vi "OCR Player2 DeleteMe.vi"(7 "error in":errorcluster) -> (27 "error out":errorcluster)   [LabVIEW 2015]
uses:
  <vilib>/vision/NI_Vision_Development_Module.lvlib
panel:
  out "Image Out":T1(plugin-control)
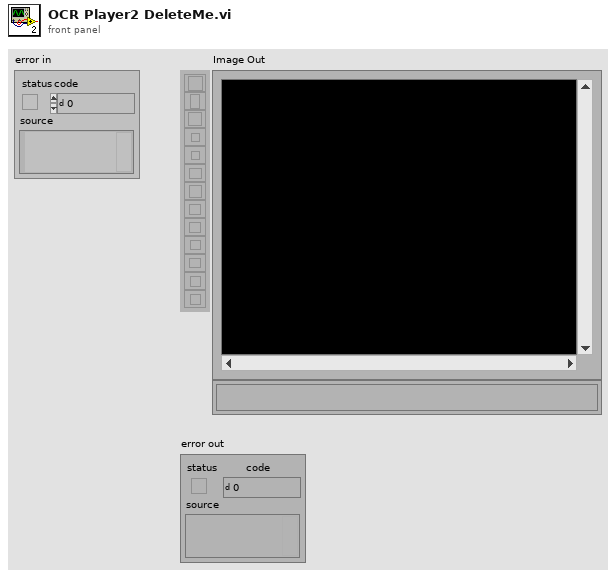
[diagram p1: front panel]
types:
  T1 = typedef "IMAQ Image.ctl" = refnum<image>
  T2 = cluster{"Threshold Data":cluster{"Method":enum16{"Fixed Range", "Uniform", "Linear", "Non Linear", "Local", "Color"}, "Looking for":u32, "Color Mode":u32, "Kernel Size":cluster{"Width":i32, "Height":i32}, "Ranges":cluster{"Min":i32, "Max":i32}[]}, "Reject Border":bool, "Number Of Erosions":i32, "Size & Spacing":cluster{"Segment Algorithm":u16, "Min Bounding Rect Width":i32, "Max Bounding Rect Width":i32, "Min Bounding Rect Height":i32, "Max Bounding Rect Height":i32, "Min Character Size":i32, "Max Character Size":i32, "Min Char Spacing":i32, "Max Horiz Element Spacing":i32, "Max Vert Element Spacing":i32, "Max Space Distance":i32}, "Read Options":cluster{"Read Strategy":i32, "Read Resolution":i32, "Scale Dependant":bool, "Aspect Ratio":i32, "Acceptance Level":i32, "Substitution Character":string, "MultiLine":bool}, "Valid Characters":cluster{"Pre-defined characters":i32, "User-defined characters":string}[], "Use Text Pattern":bool, "Orientation":u32, "# Lines Expected":u32, "Number of Blocks":i32}
  T3 = cluster{"Global Rectangle":i32[], "Contours":cluster{"ID":enum32{"External", "Internal"}, "Type":u32, "Coordinates":i32[]}[]}
  T4 = typedef "Image Type" = u32
  T5 = typedef "IMAQ OCR Session.ctl" = refnum<k1>
diagram:
  w1 = u32 0 items=["Grayscale", "Binary", "Gradient", "Rainbow", "Temperature", "User Defined", "Binary 16 Bit", "Gradient 16 Bit", "Rainbow 16 Bit", "Temperature 16 Bit", "User Defined 16 Bit"] ("Palette Type")
  w10 = T2 {"Threshold Data"={"Method"=enum."Uniform", "Looking for"=1, "Color Mode"=0, "Kernel Size"={"Width"=32, "Height"=32}, "Ranges"=[{"Min"=1, "Max"=255}]}, "Reject Border"=TRUE, "Number Of Erosions"=0, "Size & Spacing"={"Segment Algorithm"=0, "Min Bounding Rect Width"=2, "Max Bounding Rect Width"=8, "Min Bounding Rect Height"=2, "Max Bounding Rect Height"=65536, "Min Character Size"=4, "Max Character Size"=5555, "Min Char Spacing"=1, "Max Horiz Element Spacing"=1, "Max Vert Element Spacing"=0, "Max Space Distance"=65536}, "Read Options"={"Read Strategy"=1, "Read Resolution"=2, "Scale Dependant"=FALSE, "Aspect Ratio"=400, "Acceptance Level"=700, "Substitution Character"="?", "MultiLine"=FALSE}, "Valid Characters"=[], "Use Text Pattern"=FALSE, "Orientation"=0, "# Lines Expected"=0, "Number of Blocks"=4}  # Parameters
  w11 = T3 {"Global Rectangle"=[720, 494, 833, 510], "Contours"=[{"ID"=enum."External", "Type"=3, "Coordinates"=[720, 494, 833, 510]}]}  # ROI Descriptor
  w19 = T2 {"Threshold Data"={"Method"=enum."Uniform", "Looking for"=1, "Color Mode"=0, "Kernel Size"={"Width"=32, "Height"=32}, "Ranges"=[{"Min"=1, "Max"=255}]}, "Reject Border"=TRUE, "Number Of Erosions"=0, "Size & Spacing"={"Segment Algorithm"=0, "Min Bounding Rect Width"=2, "Max Bounding Rect Width"=8, "Min Bounding Rect Height"=2, "Max Bounding Rect Height"=65536, "Min Character Size"=4, "Max Character Size"=5555, "Min Char Spacing"=1, "Max Horiz Element Spacing"=1, "Max Vert Element Spacing"=0, "Max Space Distance"=65536}, "Read Options"={"Read Strategy"=1, "Read Resolution"=2, "Scale Dependant"=FALSE, "Aspect Ratio"=400, "Acceptance Level"=700, "Substitution Character"="?", "MultiLine"=FALSE}, "Valid Characters"=[], "Use Text Pattern"=FALSE, "Orientation"=0, "# Lines Expected"=0, "Number of Blocks"=4}  # Parameters
  w20 = T3 {"Global Rectangle"=[523, 533, 645, 550], "Contours"=[{"ID"=enum."External", "Type"=3, "Coordinates"=[523, 533, 645, 550]}]}  # ROI Descriptor
  w28 = T2 {"Threshold Data"={"Method"=enum."Uniform", "Looking for"=1, "Color Mode"=0, "Kernel Size"={"Width"=32, "Height"=32}, "Ranges"=[{"Min"=1, "Max"=255}]}, "Reject Border"=TRUE, "Number Of Erosions"=0, "Size & Spacing"={"Segment Algorithm"=0, "Min Bounding Rect Width"=2, "Max Bounding Rect Width"=8, "Min Bounding Rect Height"=2, "Max Bounding Rect Height"=65536, "Min Character Size"=4, "Max Character Size"=5555, "Min Char Spacing"=1, "Max Horiz Element Spacing"=1, "Max Vert Element Spacing"=0, "Max Space Distance"=65536}, "Read Options"={"Read Strategy"=1, "Read Resolution"=2, "Scale Dependant"=FALSE, "Aspect Ratio"=400, "Acceptance Level"=700, "Substitution Character"="?", "MultiLine"=FALSE}, "Valid Characters"=[], "Use Text Pattern"=FALSE, "Orientation"=0, "# Lines Expected"=0, "Number of Blocks"=4}  # Parameters
  w29 = T3 {"Global Rectangle"=[386, 689, 502, 706], "Contours"=[{"ID"=enum."External", "Type"=3, "Coordinates"=[386, 689, 502, 706]}]}  # ROI Descriptor
  w37 = T2 {"Threshold Data"={"Method"=enum."Uniform", "Looking for"=1, "Color Mode"=0, "Kernel Size"={"Width"=32, "Height"=32}, "Ranges"=[{"Min"=1, "Max"=255}]}, "Reject Border"=TRUE, "Number Of Erosions"=0, "Size & Spacing"={"Segment Algorithm"=0, "Min Bounding Rect Width"=2, "Max Bounding Rect Width"=8, "Min Bounding Rect Height"=2, "Max Bounding Rect Height"=65536, "Min Character Size"=4, "Max Character Size"=5555, "Min Char Spacing"=1, "Max Horiz Element Spacing"=1, "Max Vert Element Spacing"=0, "Max Space Distance"=65536}, "Read Options"={"Read Strategy"=1, "Read Resolution"=2, "Scale Dependant"=FALSE, "Aspect Ratio"=400, "Acceptance Level"=700, "Substitution Character"="?", "MultiLine"=FALSE}, "Valid Characters"=[], "Use Text Pattern"=FALSE, "Orientation"=0, "# Lines Expected"=0, "Number of Blocks"=4}  # Parameters
  w38 = T3 {"Global Rectangle"=[543, 836, 661, 852], "Contours"=[{"ID"=enum."External", "Type"=3, "Coordinates"=[543, 836, 661, 852]}]}  # ROI Descriptor
  w46 = T2 {"Threshold Data"={"Method"=enum."Uniform", "Looking for"=1, "Color Mode"=0, "Kernel Size"={"Width"=32, "Height"=32}, "Ranges"=[{"Min"=1, "Max"=255}]}, "Reject Border"=TRUE, "Number Of Erosions"=0, "Size & Spacing"={"Segment Algorithm"=0, "Min Bounding Rect Width"=2, "Max Bounding Rect Width"=8, "Min Bounding Rect Height"=2, "Max Bounding Rect Height"=65536, "Min Character Size"=4, "Max Character Size"=5555, "Min Char Spacing"=1, "Max Horiz Element Spacing"=1, "Max Vert Element Spacing"=0, "Max Space Distance"=65536}, "Read Options"={"Read Strategy"=1, "Read Resolution"=2, "Scale Dependant"=FALSE, "Aspect Ratio"=400, "Acceptance Level"=700, "Substitution Character"="?", "MultiLine"=FALSE}, "Valid Characters"=[], "Use Text Pattern"=FALSE, "Orientation"=0, "# Lines Expected"=0, "Number of Blocks"=4}  # Parameters
  w47 = T3 {"Global Rectangle"=[757, 870, 877, 885], "Contours"=[{"ID"=enum."External", "Type"=3, "Coordinates"=[757, 870, 877, 885]}]}  # ROI Descriptor
  w55 = T2 {"Threshold Data"={"Method"=enum."Uniform", "Looking for"=1, "Color Mode"=0, "Kernel Size"={"Width"=32, "Height"=32}, "Ranges"=[{"Min"=1, "Max"=255}]}, "Reject Border"=TRUE, "Number Of Erosions"=0, "Size & Spacing"={"Segment Algorithm"=0, "Min Bounding Rect Width"=2, "Max Bounding Rect Width"=8, "Min Bounding Rect Height"=2, "Max Bounding Rect Height"=65536, "Min Character Size"=4, "Max Character Size"=5555, "Min Char Spacing"=1, "Max Horiz Element Spacing"=1, "Max Vert Element Spacing"=0, "Max Space Distance"=65536}, "Read Options"={"Read Strategy"=1, "Read Resolution"=2, "Scale Dependant"=FALSE, "Aspect Ratio"=400, "Acceptance Level"=700, "Substitution Character"="?", "MultiLine"=FALSE}, "Valid Characters"=[], "Use Text Pattern"=FALSE, "Orientation"=0, "# Lines Expected"=0, "Number of Blocks"=4}  # Parameters
  w56 = T3 {"Global Rectangle"=[1029, 868, 1143, 884], "Contours"=[{"ID"=enum."External", "Type"=3, "Coordinates"=[1029, 868, 1143, 884]}]}  # ROI Descriptor
  w64 = T2 {"Threshold Data"={"Method"=enum."Uniform", "Looking for"=1, "Color Mode"=0, "Kernel Size"={"Width"=32, "Height"=32}, "Ranges"=[{"Min"=1, "Max"=255}]}, "Reject Border"=TRUE, "Number Of Erosions"=0, "Size & Spacing"={"Segment Algorithm"=0, "Min Bounding Rect Width"=2, "Max Bounding Rect Width"=8, "Min Bounding Rect Height"=2, "Max Bounding Rect Height"=65536, "Min Character Size"=4, "Max Character Size"=5555, "Min Char Spacing"=1, "Max Horiz Element Spacing"=1, "Max Vert Element Spacing"=0, "Max Space Distance"=65536}, "Read Options"={"Read Strategy"=1, "Read Resolution"=2, "Scale Dependant"=FALSE, "Aspect Ratio"=400, "Acceptance Level"=700, "Substitution Character"="?", "MultiLine"=FALSE}, "Valid Characters"=[], "Use Text Pattern"=FALSE, "Orientation"=0, "# Lines Expected"=0, "Number of Blocks"=4}  # Parameters
  w65 = T3 {"Global Rectangle"=[1264, 838, 1374, 853], "Contours"=[{"ID"=enum."External", "Type"=3, "Coordinates"=[1264, 838, 1374, 853]}]}  # ROI Descriptor
  w73 = T2 {"Threshold Data"={"Method"=enum."Uniform", "Looking for"=1, "Color Mode"=0, "Kernel Size"={"Width"=32, "Height"=32}, "Ranges"=[{"Min"=1, "Max"=255}]}, "Reject Border"=TRUE, "Number Of Erosions"=0, "Size & Spacing"={"Segment Algorithm"=0, "Min Bounding Rect Width"=2, "Max Bounding Rect Width"=8, "Min Bounding Rect Height"=2, "Max Bounding Rect Height"=65536, "Min Character Size"=4, "Max Character Size"=5555, "Min Char Spacing"=1, "Max Horiz Element Spacing"=1, "Max Vert Element Spacing"=0, "Max Space Distance"=65536}, "Read Options"={"Read Strategy"=1, "Read Resolution"=2, "Scale Dependant"=FALSE, "Aspect Ratio"=400, "Acceptance Level"=700, "Substitution Character"="?", "MultiLine"=FALSE}, "Valid Characters"=[], "Use Text Pattern"=FALSE, "Orientation"=0, "# Lines Expected"=0, "Number of Blocks"=4}  # Parameters
  w74 = T3 {"Global Rectangle"=[1385, 697, 1502, 712], "Contours"=[{"ID"=enum."External", "Type"=3, "Coordinates"=[1385, 697, 1502, 712]}]}  # ROI Descriptor
  w82 = T2 {"Threshold Data"={"Method"=enum."Uniform", "Looking for"=1, "Color Mode"=0, "Kernel Size"={"Width"=32, "Height"=32}, "Ranges"=[{"Min"=1, "Max"=255}]}, "Reject Border"=TRUE, "Number Of Erosions"=0, "Size & Spacing"={"Segment Algorithm"=0, "Min Bounding Rect Width"=2, "Max Bounding Rect Width"=8, "Min Bounding Rect Height"=2, "Max Bounding Rect Height"=65536, "Min Character Size"=4, "Max Character Size"=5555, "Min Char Spacing"=1, "Max Horiz Element Spacing"=1, "Max Vert Element Spacing"=0, "Max Space Distance"=65536}, "Read Options"={"Read Strategy"=1, "Read Resolution"=2, "Scale Dependant"=FALSE, "Aspect Ratio"=400, "Acceptance Level"=700, "Substitution Character"="?", "MultiLine"=FALSE}, "Valid Characters"=[], "Use Text Pattern"=FALSE, "Orientation"=0, "# Lines Expected"=0, "Number of Blocks"=4}  # Parameters
  w83 = T3 {"Global Rectangle"=[1249, 535, 1360, 550], "Contours"=[{"ID"=enum."External", "Type"=3, "Coordinates"=[1249, 535, 1360, 550]}]}  # ROI Descriptor
  w91 = T2 {"Threshold Data"={"Method"=enum."Uniform", "Looking for"=1, "Color Mode"=0, "Kernel Size"={"Width"=32, "Height"=32}, "Ranges"=[{"Min"=1, "Max"=255}]}, "Reject Border"=TRUE, "Number Of Erosions"=0, "Size & Spacing"={"Segment Algorithm"=0, "Min Bounding Rect Width"=2, "Max Bounding Rect Width"=8, "Min Bounding Rect Height"=2, "Max Bounding Rect Height"=65536, "Min Character Size"=4, "Max Character Size"=5555, "Min Char Spacing"=1, "Max Horiz Element Spacing"=1, "Max Vert Element Spacing"=0, "Max Space Distance"=65536}, "Read Options"={"Read Strategy"=1, "Read Resolution"=2, "Scale Dependant"=FALSE, "Aspect Ratio"=400, "Acceptance Level"=700, "Substitution Character"="?", "MultiLine"=FALSE}, "Valid Characters"=[], "Use Text Pattern"=FALSE, "Orientation"=0, "# Lines Expected"=0, "Number of Blocks"=4}  # Parameters
  w92 = T3 {"Global Rectangle"=[1068, 495, 1179, 512], "Contours"=[{"ID"=enum."External", "Type"=3, "Coordinates"=[1068, 495, 1179, 512]}]}  # ROI Descriptor
  w96 = 1 items=["Red", "Green", "Blue", "Hue", "Saturation", "Luminance", "Value", "Intensity"] ("Color Plane")
  w97 = T4 4 items=["Grayscale (U8)", "Grayscale (I16)", "Grayscale (SGL)", "Complex (CSG)", "RGB (U32)", "HSL (U32)", "RGB (U64)", "Grayscale (U16)"] ("Image Type")
  n1 = Call Chain() -> (call chain=w101:string[])
  n2 = Index Array(array=w101) -> (element=w100:string)  [unwired: 1 in]
  n3 = call "File Dialog"("prompt"="Select an image file...") -> ("selected path"=w98:path)  [unwired: 6 in, 8 out]
  n4 = call "IMAQ Create"("Image Name"=w100, "Image Type"=w97, "error in (no error)"="error in") -> ("New Image"=w104:T1, "error out"=w103:errorcluster)  [unwired: 1 in, 1 out]
  n5 = call "IMAQ ReadFile"("File Path"=w98, "error in (no error)"=w103, "Image"=w104) -> ("error out"=w105:errorcluster, "Image Out"=w95:T1)  [unwired: 2 in, 5 out]
  n6 = call "IMAQ ExtractSingleColorPlane"("Color Plane"=w96, "error in (no error)"=w105, "Image Src"=w95) -> ("error out"=w94:errorcluster, "Image Dst Out"=w2:T1)  [unwired: 1 in, 6 out]
  "Image Out" <- w2
  n7 = while "Create an OCR session and read the character set file.\nSet paramaters from Vision Assistant Step." {
    shift-right: [w110] -> w89
    shift-left: _ -> [w109]
    tunnel: w94 -> [w112]
    tunnel: w91 -> [w108]
    tunnel: path "C:/Users/Bob Dabalina/Documents/Labview/OCR Practice/Views Numbers.abc" ("File Path") -> [w107]
    tunnel: [w106] -> w90
    stop <- FALSE continue-if-true
    n8 = First Call?() -> (First Call?: T/F=w111:bool)
    n9 = case shown="True" w111 {
      tunnel: w107 -> [_ w119]
      tunnel: w112 -> [w114 w123]
      tunnel: [w115 w121] -> w110
      tunnel: [w114 w120] -> w106
      tunnel: w108 -> [_ w116]
      tunnel: w109 -> [w115 _]
      frame False {
      }
      frame True {
        w124 = 0 items=["Read All", "Read Character Set Only", "Read Properties Only"] ("Read Options")
        n10 = call <vilib>:"IVA Get Alternate Path.vi"("Path In"=w119) -> ("Path Out"=w118:path)  [unwired: 10 out]
        n11 = call "IMAQ OCR Create Session"("error in (no error)"=w123) -> ("error out"=w125:errorcluster, "IMAQ OCR Session"=w126:T5)  [unwired: 9 out]
        n12 = call "IMAQ OCR Read Character Set File"("File Path"=w118, "error in (no error)"=w125, "Read Options"=w124, "IMAQ OCR Session"=w126) -> ("error out"=w122:errorcluster, "IMAQ OCR Session (dup)"=w117:T5)  [unwired: 1 in, 5 out]
        n13 = call <vilib>:"IVA OCR - Set Parameters 2.vi"("error in (no error)"=w122, "Parameters"=w116, "IMAQ OCR Session"=w117) -> ("error out"=w120:errorcluster, "IMAQ OCR Session Out"=w121:T5)  [unwired: 7 in]
      }
    }
  }
  n14 = Unbundle By Name(w91) -> ("# Lines Expected"=w87:u32, "Orientation"=w88:u32)
  n15 = call "IMAQ OCR Read Text 4"("IMAQ OCR Session"=w89, "ROI Descriptor"=w92, "Image"=w2, "Number of Lines Requested"=w87, "error in (no error)"=w90, "Orientation"=w88) -> ("error out"=w86:errorcluster)  [unwired: 9 out]
  n16 = call <vilib>:"IVA Clear Coordsys Errors.vi"("error in (no error)"=w86) -> ("error out"=w85:errorcluster)  [unwired: 10 in]
  n17 = while "Create an OCR session and read the character set file.\nSet paramaters from Vision Assistant Step." {
    shift-right: [w131] -> w80
    shift-left: _ -> [w130]
    tunnel: w85 -> [w133]
    tunnel: w82 -> [w129]
    tunnel: path "C:/Users/Bob Dabalina/Documents/Labview/OCR Practice/Views Numbers.abc" ("File Path") -> [w128]
    tunnel: [w127] -> w81
    stop <- FALSE continue-if-true
    n18 = First Call?() -> (First Call?: T/F=w132:bool)
    n19 = case shown="True" w132 {
      tunnel: w128 -> [_ w140]
      tunnel: w133 -> [w135 w144]
      tunnel: [w136 w142] -> w131
      tunnel: [w135 w141] -> w127
      tunnel: w129 -> [_ w137]
      tunnel: w130 -> [w136 _]
      frame False {
      }
      frame True {
        w145 = 0 items=["Read All", "Read Character Set Only", "Read Properties Only"] ("Read Options")
        n20 = call <vilib>:"IVA Get Alternate Path.vi"("Path In"=w140) -> ("Path Out"=w139:path)  [unwired: 10 out]
        n21 = call "IMAQ OCR Create Session"("error in (no error)"=w144) -> ("error out"=w146:errorcluster, "IMAQ OCR Session"=w147:T5)  [unwired: 9 out]
        n22 = call "IMAQ OCR Read Character Set File"("File Path"=w139, "error in (no error)"=w146, "Read Options"=w145, "IMAQ OCR Session"=w147) -> ("error out"=w143:errorcluster, "IMAQ OCR Session (dup)"=w138:T5)  [unwired: 1 in, 5 out]
        n23 = call <vilib>:"IVA OCR - Set Parameters 2.vi"("error in (no error)"=w143, "Parameters"=w137, "IMAQ OCR Session"=w138) -> ("error out"=w141:errorcluster, "IMAQ OCR Session Out"=w142:T5)  [unwired: 7 in]
      }
    }
  }
  n24 = Unbundle By Name(w82) -> ("# Lines Expected"=w78:u32, "Orientation"=w79:u32)
  n25 = call "IMAQ OCR Read Text 4"("IMAQ OCR Session"=w80, "ROI Descriptor"=w83, "Image"=w2, "Number of Lines Requested"=w78, "error in (no error)"=w81, "Orientation"=w79) -> ("error out"=w77:errorcluster)  [unwired: 9 out]
  n26 = call <vilib>:"IVA Clear Coordsys Errors.vi"("error in (no error)"=w77) -> ("error out"=w76:errorcluster)  [unwired: 10 in]
  n27 = while "Create an OCR session and read the character set file.\nSet paramaters from Vision Assistant Step." {
    shift-right: [w152] -> w71
    shift-left: _ -> [w151]
    tunnel: w76 -> [w154]
    tunnel: w73 -> [w150]
    tunnel: path "C:/Users/Bob Dabalina/Documents/Labview/OCR Practice/Views Numbers.abc" ("File Path") -> [w149]
    tunnel: [w148] -> w72
    stop <- FALSE continue-if-true
    n28 = First Call?() -> (First Call?: T/F=w153:bool)
    n29 = case shown="True" w153 {
      tunnel: w149 -> [_ w161]
      tunnel: w154 -> [w156 w165]
      tunnel: [w157 w163] -> w152
      tunnel: [w156 w162] -> w148
      tunnel: w150 -> [_ w158]
      tunnel: w151 -> [w157 _]
      frame False {
      }
      frame True {
        w166 = 0 items=["Read All", "Read Character Set Only", "Read Properties Only"] ("Read Options")
        n30 = call <vilib>:"IVA Get Alternate Path.vi"("Path In"=w161) -> ("Path Out"=w160:path)  [unwired: 10 out]
        n31 = call "IMAQ OCR Create Session"("error in (no error)"=w165) -> ("error out"=w167:errorcluster, "IMAQ OCR Session"=w168:T5)  [unwired: 9 out]
        n32 = call "IMAQ OCR Read Character Set File"("File Path"=w160, "error in (no error)"=w167, "Read Options"=w166, "IMAQ OCR Session"=w168) -> ("error out"=w164:errorcluster, "IMAQ OCR Session (dup)"=w159:T5)  [unwired: 1 in, 5 out]
        n33 = call <vilib>:"IVA OCR - Set Parameters 2.vi"("error in (no error)"=w164, "Parameters"=w158, "IMAQ OCR Session"=w159) -> ("error out"=w162:errorcluster, "IMAQ OCR Session Out"=w163:T5)  [unwired: 7 in]
      }
    }
  }
  n34 = Unbundle By Name(w73) -> ("# Lines Expected"=w69:u32, "Orientation"=w70:u32)
  n35 = call "IMAQ OCR Read Text 4"("IMAQ OCR Session"=w71, "ROI Descriptor"=w74, "Image"=w2, "Number of Lines Requested"=w69, "error in (no error)"=w72, "Orientation"=w70) -> ("error out"=w68:errorcluster)  [unwired: 9 out]
  n36 = call <vilib>:"IVA Clear Coordsys Errors.vi"("error in (no error)"=w68) -> ("error out"=w67:errorcluster)  [unwired: 10 in]
  n37 = while "Create an OCR session and read the character set file.\nSet paramaters from Vision Assistant Step." {
    shift-right: [w173] -> w62
    shift-left: _ -> [w172]
    tunnel: w67 -> [w175]
    tunnel: w64 -> [w171]
    tunnel: path "C:/Users/Bob Dabalina/Documents/Labview/OCR Practice/Views Numbers.abc" ("File Path") -> [w170]
    tunnel: [w169] -> w63
    stop <- FALSE continue-if-true
    n38 = First Call?() -> (First Call?: T/F=w174:bool)
    n39 = case shown="True" w174 {
      tunnel: w170 -> [_ w182]
      tunnel: w175 -> [w177 w186]
      tunnel: [w178 w184] -> w173
      tunnel: [w177 w183] -> w169
      tunnel: w171 -> [_ w179]
      tunnel: w172 -> [w178 _]
      frame False {
      }
      frame True {
        w187 = 0 items=["Read All", "Read Character Set Only", "Read Properties Only"] ("Read Options")
        n40 = call <vilib>:"IVA Get Alternate Path.vi"("Path In"=w182) -> ("Path Out"=w181:path)  [unwired: 10 out]
        n41 = call "IMAQ OCR Create Session"("error in (no error)"=w186) -> ("error out"=w188:errorcluster, "IMAQ OCR Session"=w189:T5)  [unwired: 9 out]
        n42 = call "IMAQ OCR Read Character Set File"("File Path"=w181, "error in (no error)"=w188, "Read Options"=w187, "IMAQ OCR Session"=w189) -> ("error out"=w185:errorcluster, "IMAQ OCR Session (dup)"=w180:T5)  [unwired: 1 in, 5 out]
        n43 = call <vilib>:"IVA OCR - Set Parameters 2.vi"("error in (no error)"=w185, "Parameters"=w179, "IMAQ OCR Session"=w180) -> ("error out"=w183:errorcluster, "IMAQ OCR Session Out"=w184:T5)  [unwired: 7 in]
      }
    }
  }
  n44 = Unbundle By Name(w64) -> ("# Lines Expected"=w60:u32, "Orientation"=w61:u32)
  n45 = call "IMAQ OCR Read Text 4"("IMAQ OCR Session"=w62, "ROI Descriptor"=w65, "Image"=w2, "Number of Lines Requested"=w60, "error in (no error)"=w63, "Orientation"=w61) -> ("error out"=w59:errorcluster)  [unwired: 9 out]
  n46 = call <vilib>:"IVA Clear Coordsys Errors.vi"("error in (no error)"=w59) -> ("error out"=w58:errorcluster)  [unwired: 10 in]
  n47 = while "Create an OCR session and read the character set file.\nSet paramaters from Vision Assistant Step." {
    shift-right: [w194] -> w53
    shift-left: _ -> [w193]
    tunnel: w58 -> [w196]
    tunnel: w55 -> [w192]
    tunnel: path "C:/Users/Bob Dabalina/Documents/Labview/OCR Practice/Views Numbers.abc" ("File Path") -> [w191]
    tunnel: [w190] -> w54
    stop <- FALSE continue-if-true
    n48 = First Call?() -> (First Call?: T/F=w195:bool)
    n49 = case shown="True" w195 {
      tunnel: w191 -> [_ w203]
      tunnel: w196 -> [w198 w207]
      tunnel: [w199 w205] -> w194
      tunnel: [w198 w204] -> w190
      tunnel: w192 -> [_ w200]
      tunnel: w193 -> [w199 _]
      frame False {
      }
      frame True {
        w208 = 0 items=["Read All", "Read Character Set Only", "Read Properties Only"] ("Read Options")
        n50 = call <vilib>:"IVA Get Alternate Path.vi"("Path In"=w203) -> ("Path Out"=w202:path)  [unwired: 10 out]
        n51 = call "IMAQ OCR Create Session"("error in (no error)"=w207) -> ("error out"=w209:errorcluster, "IMAQ OCR Session"=w210:T5)  [unwired: 9 out]
        n52 = call "IMAQ OCR Read Character Set File"("File Path"=w202, "error in (no error)"=w209, "Read Options"=w208, "IMAQ OCR Session"=w210) -> ("error out"=w206:errorcluster, "IMAQ OCR Session (dup)"=w201:T5)  [unwired: 1 in, 5 out]
        n53 = call <vilib>:"IVA OCR - Set Parameters 2.vi"("error in (no error)"=w206, "Parameters"=w200, "IMAQ OCR Session"=w201) -> ("error out"=w204:errorcluster, "IMAQ OCR Session Out"=w205:T5)  [unwired: 7 in]
      }
    }
  }
  n54 = Unbundle By Name(w55) -> ("# Lines Expected"=w51:u32, "Orientation"=w52:u32)
  n55 = call "IMAQ OCR Read Text 4"("IMAQ OCR Session"=w53, "ROI Descriptor"=w56, "Image"=w2, "Number of Lines Requested"=w51, "error in (no error)"=w54, "Orientation"=w52) -> ("error out"=w50:errorcluster)  [unwired: 9 out]
  n56 = call <vilib>:"IVA Clear Coordsys Errors.vi"("error in (no error)"=w50) -> ("error out"=w49:errorcluster)  [unwired: 10 in]
  n57 = while "Create an OCR session and read the character set file.\nSet paramaters from Vision Assistant Step." {
    shift-right: [w215] -> w44
    shift-left: _ -> [w214]
    tunnel: w49 -> [w217]
    tunnel: w46 -> [w213]
    tunnel: path "C:/Users/Bob Dabalina/Documents/Labview/OCR Practice/Views Numbers.abc" ("File Path") -> [w212]
    tunnel: [w211] -> w45
    stop <- FALSE continue-if-true
    n58 = First Call?() -> (First Call?: T/F=w216:bool)
    n59 = case shown="True" w216 {
      tunnel: w212 -> [_ w224]
      tunnel: w217 -> [w219 w228]
      tunnel: [w220 w226] -> w215
      tunnel: [w219 w225] -> w211
      tunnel: w213 -> [_ w221]
      tunnel: w214 -> [w220 _]
      frame False {
      }
      frame True {
        w229 = 0 items=["Read All", "Read Character Set Only", "Read Properties Only"] ("Read Options")
        n60 = call <vilib>:"IVA Get Alternate Path.vi"("Path In"=w224) -> ("Path Out"=w223:path)  [unwired: 10 out]
        n61 = call "IMAQ OCR Create Session"("error in (no error)"=w228) -> ("error out"=w230:errorcluster, "IMAQ OCR Session"=w231:T5)  [unwired: 9 out]
        n62 = call "IMAQ OCR Read Character Set File"("File Path"=w223, "error in (no error)"=w230, "Read Options"=w229, "IMAQ OCR Session"=w231) -> ("error out"=w227:errorcluster, "IMAQ OCR Session (dup)"=w222:T5)  [unwired: 1 in, 5 out]
        n63 = call <vilib>:"IVA OCR - Set Parameters 2.vi"("error in (no error)"=w227, "Parameters"=w221, "IMAQ OCR Session"=w222) -> ("error out"=w225:errorcluster, "IMAQ OCR Session Out"=w226:T5)  [unwired: 7 in]
      }
    }
  }
  n64 = Unbundle By Name(w46) -> ("# Lines Expected"=w42:u32, "Orientation"=w43:u32)
  n65 = call "IMAQ OCR Read Text 4"("IMAQ OCR Session"=w44, "ROI Descriptor"=w47, "Image"=w2, "Number of Lines Requested"=w42, "error in (no error)"=w45, "Orientation"=w43) -> ("error out"=w41:errorcluster)  [unwired: 9 out]
  n66 = call <vilib>:"IVA Clear Coordsys Errors.vi"("error in (no error)"=w41) -> ("error out"=w40:errorcluster)  [unwired: 10 in]
  n67 = while "Create an OCR session and read the character set file.\nSet paramaters from Vision Assistant Step." {
    shift-right: [w236] -> w35
    shift-left: _ -> [w235]
    tunnel: w40 -> [w238]
    tunnel: w37 -> [w234]
    tunnel: path "C:/Users/Bob Dabalina/Documents/Labview/OCR Practice/Views Numbers.abc" ("File Path") -> [w233]
    tunnel: [w232] -> w36
    stop <- FALSE continue-if-true
    n68 = First Call?() -> (First Call?: T/F=w237:bool)
    n69 = case shown="True" w237 {
      tunnel: w233 -> [_ w245]
      tunnel: w238 -> [w240 w249]
      tunnel: [w241 w247] -> w236
      tunnel: [w240 w246] -> w232
      tunnel: w234 -> [_ w242]
      tunnel: w235 -> [w241 _]
      frame False {
      }
      frame True {
        w250 = 0 items=["Read All", "Read Character Set Only", "Read Properties Only"] ("Read Options")
        n70 = call <vilib>:"IVA Get Alternate Path.vi"("Path In"=w245) -> ("Path Out"=w244:path)  [unwired: 10 out]
        n71 = call "IMAQ OCR Create Session"("error in (no error)"=w249) -> ("error out"=w251:errorcluster, "IMAQ OCR Session"=w252:T5)  [unwired: 9 out]
        n72 = call "IMAQ OCR Read Character Set File"("File Path"=w244, "error in (no error)"=w251, "Read Options"=w250, "IMAQ OCR Session"=w252) -> ("error out"=w248:errorcluster, "IMAQ OCR Session (dup)"=w243:T5)  [unwired: 1 in, 5 out]
        n73 = call <vilib>:"IVA OCR - Set Parameters 2.vi"("error in (no error)"=w248, "Parameters"=w242, "IMAQ OCR Session"=w243) -> ("error out"=w246:errorcluster, "IMAQ OCR Session Out"=w247:T5)  [unwired: 7 in]
      }
    }
  }
  n74 = Unbundle By Name(w37) -> ("# Lines Expected"=w33:u32, "Orientation"=w34:u32)
  n75 = call "IMAQ OCR Read Text 4"("IMAQ OCR Session"=w35, "ROI Descriptor"=w38, "Image"=w2, "Number of Lines Requested"=w33, "error in (no error)"=w36, "Orientation"=w34) -> ("error out"=w32:errorcluster)  [unwired: 9 out]
  n76 = call <vilib>:"IVA Clear Coordsys Errors.vi"("error in (no error)"=w32) -> ("error out"=w31:errorcluster)  [unwired: 10 in]
  n77 = while "Create an OCR session and read the character set file.\nSet paramaters from Vision Assistant Step." {
    shift-right: [w257] -> w26
    shift-left: _ -> [w256]
    tunnel: w31 -> [w259]
    tunnel: w28 -> [w255]
    tunnel: path "C:/Users/Bob Dabalina/Documents/Labview/OCR Practice/Views Numbers.abc" ("File Path") -> [w254]
    tunnel: [w253] -> w27
    stop <- FALSE continue-if-true
    n78 = First Call?() -> (First Call?: T/F=w258:bool)
    n79 = case shown="True" w258 {
      tunnel: w254 -> [_ w266]
      tunnel: w259 -> [w261 w270]
      tunnel: [w262 w268] -> w257
      tunnel: [w261 w267] -> w253
      tunnel: w255 -> [_ w263]
      tunnel: w256 -> [w262 _]
      frame False {
      }
      frame True {
        w271 = 0 items=["Read All", "Read Character Set Only", "Read Properties Only"] ("Read Options")
        n80 = call <vilib>:"IVA Get Alternate Path.vi"("Path In"=w266) -> ("Path Out"=w265:path)  [unwired: 10 out]
        n81 = call "IMAQ OCR Create Session"("error in (no error)"=w270) -> ("error out"=w272:errorcluster, "IMAQ OCR Session"=w273:T5)  [unwired: 9 out]
        n82 = call "IMAQ OCR Read Character Set File"("File Path"=w265, "error in (no error)"=w272, "Read Options"=w271, "IMAQ OCR Session"=w273) -> ("error out"=w269:errorcluster, "IMAQ OCR Session (dup)"=w264:T5)  [unwired: 1 in, 5 out]
        n83 = call <vilib>:"IVA OCR - Set Parameters 2.vi"("error in (no error)"=w269, "Parameters"=w263, "IMAQ OCR Session"=w264) -> ("error out"=w267:errorcluster, "IMAQ OCR Session Out"=w268:T5)  [unwired: 7 in]
      }
    }
  }
  n84 = Unbundle By Name(w28) -> ("# Lines Expected"=w24:u32, "Orientation"=w25:u32)
  n85 = call "IMAQ OCR Read Text 4"("IMAQ OCR Session"=w26, "ROI Descriptor"=w29, "Image"=w2, "Number of Lines Requested"=w24, "error in (no error)"=w27, "Orientation"=w25) -> ("error out"=w23:errorcluster)  [unwired: 9 out]
  n86 = call <vilib>:"IVA Clear Coordsys Errors.vi"("error in (no error)"=w23) -> ("error out"=w22:errorcluster)  [unwired: 10 in]
  n87 = while "Create an OCR session and read the character set file.\nSet paramaters from Vision Assistant Step." {
    shift-right: [w278] -> w17
    shift-left: _ -> [w277]
    tunnel: w22 -> [w280]
    tunnel: w19 -> [w276]
    tunnel: path "C:/Users/Bob Dabalina/Documents/Labview/OCR Practice/Views Numbers.abc" ("File Path") -> [w275]
    tunnel: [w274] -> w18
    stop <- FALSE continue-if-true
    n88 = First Call?() -> (First Call?: T/F=w279:bool)
    n89 = case shown="True" w279 {
      tunnel: w275 -> [_ w287]
      tunnel: w280 -> [w282 w291]
      tunnel: [w283 w289] -> w278
      tunnel: [w282 w288] -> w274
      tunnel: w276 -> [_ w284]
      tunnel: w277 -> [w283 _]
      frame False {
      }
      frame True {
        w292 = 0 items=["Read All", "Read Character Set Only", "Read Properties Only"] ("Read Options")
        n90 = call <vilib>:"IVA Get Alternate Path.vi"("Path In"=w287) -> ("Path Out"=w286:path)  [unwired: 10 out]
        n91 = call "IMAQ OCR Create Session"("error in (no error)"=w291) -> ("error out"=w293:errorcluster, "IMAQ OCR Session"=w294:T5)  [unwired: 9 out]
        n92 = call "IMAQ OCR Read Character Set File"("File Path"=w286, "error in (no error)"=w293, "Read Options"=w292, "IMAQ OCR Session"=w294) -> ("error out"=w290:errorcluster, "IMAQ OCR Session (dup)"=w285:T5)  [unwired: 1 in, 5 out]
        n93 = call <vilib>:"IVA OCR - Set Parameters 2.vi"("error in (no error)"=w290, "Parameters"=w284, "IMAQ OCR Session"=w285) -> ("error out"=w288:errorcluster, "IMAQ OCR Session Out"=w289:T5)  [unwired: 7 in]
      }
    }
  }
  n94 = Unbundle By Name(w19) -> ("# Lines Expected"=w15:u32, "Orientation"=w16:u32)
  n95 = call "IMAQ OCR Read Text 4"("IMAQ OCR Session"=w17, "ROI Descriptor"=w20, "Image"=w2, "Number of Lines Requested"=w15, "error in (no error)"=w18, "Orientation"=w16) -> ("error out"=w14:errorcluster)  [unwired: 9 out]
  n96 = call <vilib>:"IVA Clear Coordsys Errors.vi"("error in (no error)"=w14) -> ("error out"=w13:errorcluster)  [unwired: 10 in]
  n97 = while "Create an OCR session and read the character set file.\nSet paramaters from Vision Assistant Step." {
    shift-right: [w299] -> w8
    shift-left: _ -> [w298]
    tunnel: w13 -> [w301]
    tunnel: w10 -> [w297]
    tunnel: path "C:/Users/Bob Dabalina/Documents/Labview/OCR Practice/Views Numbers.abc" ("File Path") -> [w296]
    tunnel: [w295] -> w9
    stop <- FALSE continue-if-true
    n98 = First Call?() -> (First Call?: T/F=w300:bool)
    n99 = case shown="True" w300 {
      tunnel: w296 -> [_ w308]
      tunnel: w301 -> [w303 w312]
      tunnel: [w304 w310] -> w299
      tunnel: [w303 w309] -> w295
      tunnel: w297 -> [_ w305]
      tunnel: w298 -> [w304 _]
      frame False {
      }
      frame True {
        w313 = 0 items=["Read All", "Read Character Set Only", "Read Properties Only"] ("Read Options")
        n100 = call <vilib>:"IVA Get Alternate Path.vi"("Path In"=w308) -> ("Path Out"=w307:path)  [unwired: 10 out]
        n101 = call "IMAQ OCR Create Session"("error in (no error)"=w312) -> ("error out"=w314:errorcluster, "IMAQ OCR Session"=w315:T5)  [unwired: 9 out]
        n102 = call "IMAQ OCR Read Character Set File"("File Path"=w307, "error in (no error)"=w314, "Read Options"=w313, "IMAQ OCR Session"=w315) -> ("error out"=w311:errorcluster, "IMAQ OCR Session (dup)"=w306:T5)  [unwired: 1 in, 5 out]
        n103 = call <vilib>:"IVA OCR - Set Parameters 2.vi"("error in (no error)"=w311, "Parameters"=w305, "IMAQ OCR Session"=w306) -> ("error out"=w309:errorcluster, "IMAQ OCR Session Out"=w310:T5)  [unwired: 7 in]
      }
    }
  }
  n104 = Unbundle By Name(w10) -> ("# Lines Expected"=w6:u32, "Orientation"=w7:u32)
  n105 = call "IMAQ OCR Read Text 4"("IMAQ OCR Session"=w8, "ROI Descriptor"=w11, "Image"=w2, "Number of Lines Requested"=w6, "error in (no error)"=w9, "Orientation"=w7) -> ("error out"=w5:errorcluster)  [unwired: 9 out]
  n106 = call <vilib>:"IVA Clear Coordsys Errors.vi"("error in (no error)"=w5) -> ("error out"=w4:errorcluster)  [unwired: 10 in]
  n107 = property on="Image Out" class="ImageControl"(error in=w4, "Palette:Palette Type"=w1) -> (error out=→"error out":errorcluster)  [unwired: 1 in, 1 out]
